vi "Handle Pre Launch Init.vi"(8 "error in (no error)":errorcluster, 11 "Transfer Line in":refnum<class "Transfer Line.lvclass">) -> (0 "error out":errorcluster, 3 "Transfer Line out":refnum<class "Transfer Line.lvclass">)   [LabVIEW 2015, in "cRIO-Carbondioxide.lvlib" / "CO2-Actor.lvlib" / "Transfer Line.lvclass"]
uses:
  Transfer Line.lvclass
  CO2 Actor Messages/Timeout Msg/Timeout Msg.lvclass
  <vilib>/ActorFramework/Message Enqueuer/Message Priority.ctl
  Controls/Sample Line State Enumerator.ctl
  Transfer Line.lvclass/Transfer Line.ctl
  subs/Sample/Sample.lvclass/Sample.ctl
  <vilib>/ActorFramework/Actor/Actor.lvclass/Actor.ctl
  <vilib>/ActorFramework/Message Enqueuer/Message Enqueuer.lvclass/Message Enqueuer.ctl
  <vilib>/ActorFramework/Actor/Read Self Enqueuer.vi
  <vilib>/ActorFramework/Message Enqueuer/Init from Existing Queue.vi
  <vilib>/ActorFramework/Actor/Actor.lvclass
  <vilib>/ActorFramework/Message Enqueuer/Message Enqueuer.lvclass
  CO2 Actor/CO2 Actor.lvclass
  subs/Sample/Sample.lvclass
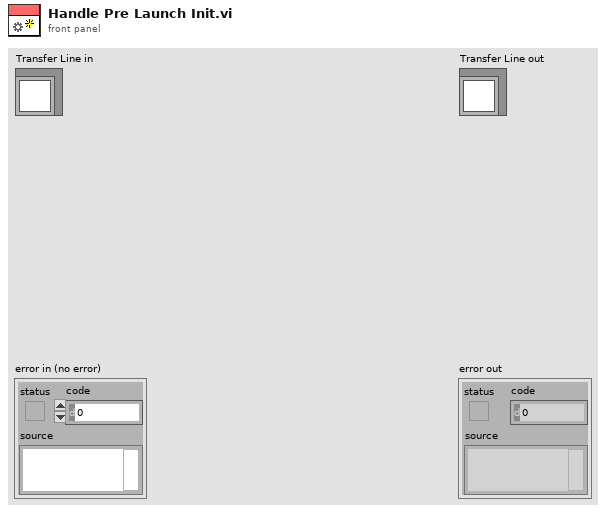
[diagram p1: front panel]
types:
  T1 = typedef "Sample Line State Enumerator.ctl" = enum16{"All lines closed", "Sample line 1.", "Sample line 2.", "Sample line 3.", "Sample line 4.", "Sample line 5.", "Out of range"}
  T2 = cluster{"Read Access":enum8{"Allowed", "Required", "None"}, "Write Access":enum8{"Allowed", "Required", "None"}}
  T3 = typedef "Actor Framework.lvlib/Message Enqueuer.lvclass/Message Priority.ctl" = enum16{"Low", "Normal", "High"}
  T4 = typedef "Sample Container.ctl" = cluster{"Sample In":refnum<k21>, "Sample Name":refnum<k21>, "Ti Cathode":refnum<k21>, "SampleQ":refnum<queue>}
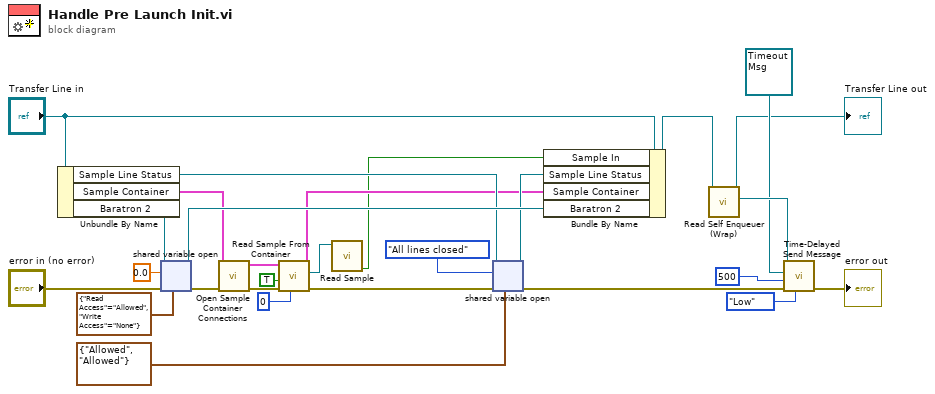
[diagram p0: block diagram]
diagram:
  n1 = Unbundle By Name("Transfer Line in") -> ("Sample Line Status"=w18:refnum<k21>, "Sample Container"=w20:T4, "Baratron 2"=w22:refnum<k21>)
  n2 = shared-variable-open(w22, "error in (no error)", 0.0, T2 {"Read Access"=enum."Allowed", "Write Access"=enum."None"} ("access")) -> (w21:refnum<k21>, w13:errorcluster)
  n3 = call "Open Sample Container Connections.vi"("error in (no error)"=w13, "Container in"=w20) -> ("error out"=w8:errorcluster, "Container out"=w5:T4)  [unwired: 8 in]
  n4 = call "Read Sample From Container.vi"("Queue timeout in ms (-1)"=0, "error in (no error)"=w8, "Read from SHV (F)"=TRUE, "Container"=w5) -> ("error out"=w6:errorcluster, "Sample out"=w3:refnum<class "Sample.lvclass">, "Container"=w4:T4)  [unwired: 3 in, 2 out]
  n5 = call "Read Sample.vi"("Sample in"=w3) -> ("Sample In"=w2:bool)  [unwired: 6 in, 4 out]
  n6 = shared-variable-open(w18, w6, Sample_Line_State_Enumerator."All lines closed" ("Enum"), T2 {"Read Access"=enum."Allowed", "Write Access"=enum."Allowed"} ("access")) -> (w16:refnum<k21>, w19:errorcluster)
  n7 = Bundle By Name(cluster="Transfer Line in", "Sample In"=w2, "Sample Line Status"=w16, "Sample Container"=w4, "Baratron 2"=w21) -> (w24:refnum<class "Transfer Line.lvclass">)
  n8 = call "Read Self Enqueuer (Wrap).vi"("CO2 Actor in"=w24) -> ("Actor Framework:Message Enqueuer"=w28:refnum<class "Message Enqueuer.lvclass">, "CO2 Actor out"=→"Transfer Line out":refnum<class "Transfer Line.lvclass">)  [unwired: 9 in]
  n9 = call <vilib>:"Time-Delayed Send Message.vi"("Message Priority (Normal)"=Message_Priority."Low", "error in (no error)"=w19, "Milliseconds To Wait"=500, "Message"=refnum<class "Timeout Msg.lvclass"> refnum ("Timeout Msg.lvclass"), "Message Enqueuer"=w28) -> ("error out"=→"error out":errorcluster)  [unwired: 5 in, 1 out]
